vi "Set Output Voltages.vi"(8 "Error In":errorcluster, 10 "Voltages":dbl[unit][](array[numeric]), 11 "BNT_DAQmx-MCSV in":refnum<class "BNT_DAQmx-MCSV.lvclass">) -> (0 "Error Out":errorcluster, 3 "BNT_DAQmx-MCSV out":refnum<class "BNT_DAQmx-MCSV.lvclass">)   [LabVIEW 2016, in "BNT_DAQmx.lvlib" / "BNT_DAQmx-MCSV.lvclass"]
doc: "Write voltage values to DAQmx device and publish.\n\nTimeout is set to constant 1s."
uses:
  BNT_DAQmx-MCSV.lvclass
  BNT_DAQmx-MCSV.lvclass/BNT_DAQmx-MCSV.ctl
  CSPP_Core/Classes/CS++ProcessVariables/PVConnection/PVConnection.lvclass/PVConnection.ctl
  CSPP_Core/Classes/CS++ProcessVariables/ProcessVariable/PV.lvclass/PV.ctl
  <vilib>/DAQmx/write.llb/DAQmx Write (Analog 1D DBL NChan 1Samp).vi
  CSPP_Core/Classes/CS++ProcessVariables/ProcessVariable/Write Data.vi
  CSPP_Core/Classes/CS++ProcessVariables/ProcessVariable/Write Error.vi
  CSPP_Core/Classes/CS++ProcessVariables/ProcessVariable/Write Quality.vi
  CSPP_Core/Classes/CS++ProcessVariables/ProcessVariable/Write status.vi
  CSPP_Core/Classes/CS++ProcessVariables/ProcessVariable/Write Timestamp.vi
  <vilib>/DAQmx/miscellaneous.llb/DAQmx Fill In Error Info.vi
  CSPP_Core/Classes/CS++ProcessVariables/ProcessVariable/PV.lvclass
  CSPP_Core/Classes/CS++ProcessVariables/PVConnection/PVConnection.lvclass
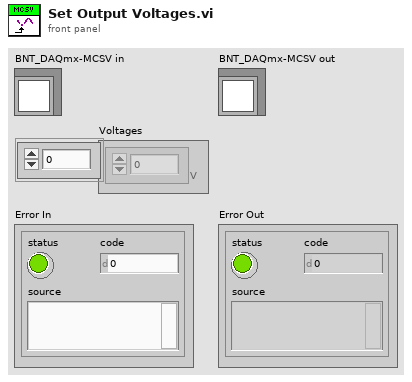
[diagram p1: front panel]
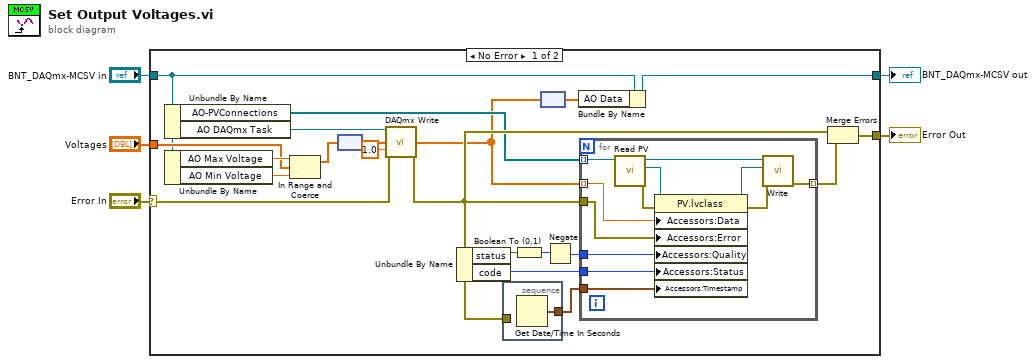
[diagram p0: block diagram]
diagram:
  n1 = case shown="No Error" "Error In" {
    selector: "Error In" -> [w23 w40]
    tunnel: [w15 w40] -> w4
    tunnel: [w6 w39] -> w2
    tunnel: "BNT_DAQmx-MCSV in" -> [w7 w39]
    tunnel: "Voltages" -> [w11 _]
    frame No Error {
      n2 = Unbundle By Name(w7) -> ("AO-PVConnections"=w14:refnum<class "PVConnection.lvclass">[], "AO DAQmx Task"=w25:refnum<k21>)
      n3 = Unbundle By Name(w7) -> ("AO Max Voltage"=w13:dbl[unit], "AO Min Voltage"=w12:dbl[unit])
      n4 = In Range and Coerce(upper limit=w13, x=w11, lower limit=w12) -> (coerced(x)=w10:dbl[unit][])  [unwired: 1 out]
      n5 = node(w10) -> (w9:dbl[])
      n6 = call-poly <vilib>:"DAQmx Write.vi"("task/channels in"=w25, "data"=w9, "timeout"=1.0, "error in"=w23) -> ("error out"=w16:errorcluster)  [unwired: 9 in, 2 out]
      n7 = Unbundle By Name(w16) -> ("status"=w18:bool, "code"=w21:i32)
      n8 = stacked-sequence {
        tunnel: [w26] -> w22
        tunnel: w16 -> [_]
        frame #0 {
          n9 = Get Date/Time In Seconds() -> (seconds since 1Jan1904=w26:timestamp)
        }
      }
      n10 = Boolean To (0,1)(Boolean=w18) -> (0, 1=w19:i16)
      n11 = node(w9) -> (w8:dbl[unit][])
      n12 = Negate(x=w19) -> (-x=w20:i16)
      n13 = Bundle By Name(cluster=w7, "AO Data"=w8) -> (w6:refnum<class "BNT_DAQmx-MCSV.lvclass">)
      n14 = for {
        tunnel: w14 -> [w30] mode=indexing
        tunnel: w9 -> [w38] mode=indexing
        tunnel: w16 -> [w37]
        tunnel: [w34] -> w17 mode=indexing
        tunnel: w20 -> [w33]
        tunnel: w21 -> [w32]
        tunnel: w22 -> [w31]
        n15 = call "Read PV.vi"("PVConnection in"=w30) -> ("error out"=w27:errorcluster, "PV"=w28:refnum<class "PV.lvclass">, "PVConnection out"=w29:refnum<class "PVConnection.lvclass">)  [unwired: 8 in]
        n16 = property class="PV.lvclass"(reference=w28, error in=w27, "Accessors:Data"=w38, "Accessors:Error"=w37, "Accessors:Quality"=w33, "Accessors:Status"=w32, "Accessors:Timestamp"=w31) -> (reference out=w36:refnum<class "PV.lvclass">, error out=w35:errorcluster)
        n17 = call "Write.vi"("error in (no error)"=w35, "PV"=w36, "PVConnection in"=w29) -> ("error out"=w34:errorcluster)  [unwired: 7 in, 1 out]
      }
      n18 = Merge Errors(w16, w17) -> (w15:errorcluster)
    }
    frame Error {
    }
  }
  "Error Out" <- w4
  "BNT_DAQmx-MCSV out" <- w2
